vi "Configure Over Voltage Protection.vi"(7 "Slave Address":i32=-1 min=-1 max=30 step=1, 8 "error":errorcluster, 9 "Set OVP Max":bool, 10 "OVP Level":dbl format="%.4f", 11 "VISA":refnum<visa-resource-name>) -> (0 "error out":errorcluster, 3 "VISA out":refnum<visa-resource-name>)   [LabVIEW 2025, in "TDK-Lambda GEN LAN Series.lvlib"]
doc: "Configure the Over-Voltage Protection (OVP) level. The power supply will go into an OVP fault if its output voltage exceeds this value. The OVP value must be higher than the voltage limit setting or an error is returned.\n\nIf \"Set OVP Max\" is set TRUE, the OVP Level input is ignored."
uses:
  <userlib>/TDK-Lambda GEN LAN Series/TDK-Lambda GEN LAN Series.lvlib
panel:
  # "TDK-Lambda Genesys \n   LAN\n  DC Power Supplies"
  # "Set the Over-Voltage \nProtection Level  (OVP)"
  # "(c) 2019 TDK-Lambda.  ALL RIGHTS RESERVED."
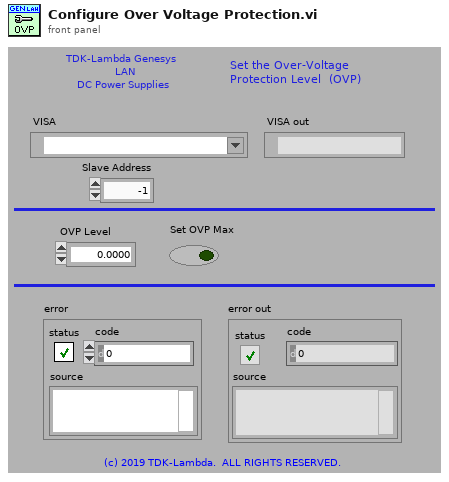
[diagram p1: front panel]
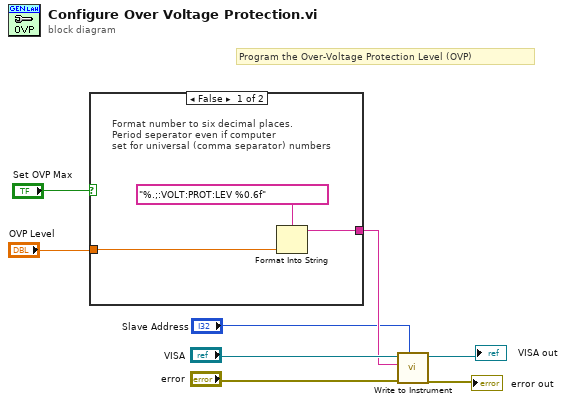
[diagram p0: block diagram]
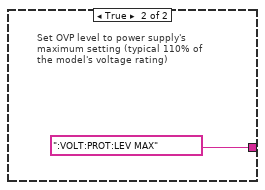
[diagram p2: hidden frame]
diagram:
  # "Program the Over-Voltage Protection Level (OVP)"
  n1 = case shown="False" "Set OVP Max" {
    tunnel: [w10 ":VOLT:PROT:LEV MAX" ("format string")] -> w5
    tunnel: "OVP Level" -> [w9 _]
    frame False {
      # "Format number to six decimal places.\nPeriod seperator even if computer \nset for universal (comma separator) numbers"
      n2 = Format Into String(format string="%.;:VOLT:PROT:LEV %0.6f", w9) -> (resulting string=w10:string)  [unwired: 2 in, 1 out]
    }
    frame True {
      # "Set OVP level to power supply's \nmaximum setting (typical 110% of\nthe model's voltage rating)"
    }
  }
  n3 = call <userlib>:"Write to Instrument.vi"("Slave Address"="Slave Address", "error"="error", "Command"=w5, "VISA"="VISA") -> ("error out"=→"error out":errorcluster, "VISA out"=→"VISA out":refnum<visa-resource-name>)  [unwired: 6 in]
